vi "Get 7280 Formated Parameters.VI"(8 "error in (no error)":errorcluster, 10 "Initial String":string, 11 "VISA Resource Name":refnum<visa-resource-name>) -> (0 "error out":errorcluster, 1 "Sensitivity":dbl format="%.4e", 2 "Frequency":dbl format="%.2e", 3 "Parameters":string, 4 "Time Constant":dbl format="%.2e", 5 "Oscillator voltage":dbl format="%.2e", 6 "Data titles":string[](array[string])=["PE7280_Vx (V)", "PE7280_Vy (V)"], 7 "VISA Resource Name Out":refnum<visa-resource-name>)   [LabVIEW 2015]
uses:
  GPIB/VISA  Send Receive.vi
panel:
  out "Ref. phase":dbl format="%.2f"
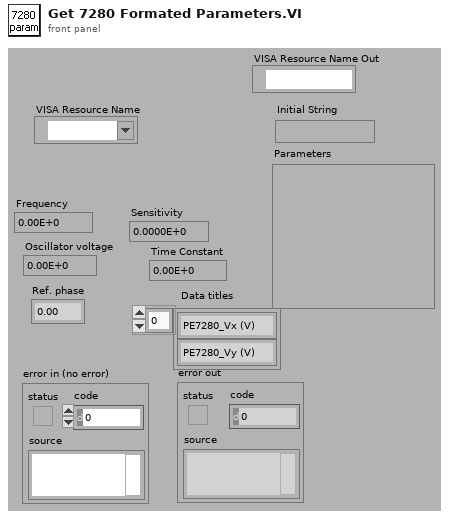
[diagram p1: front panel]
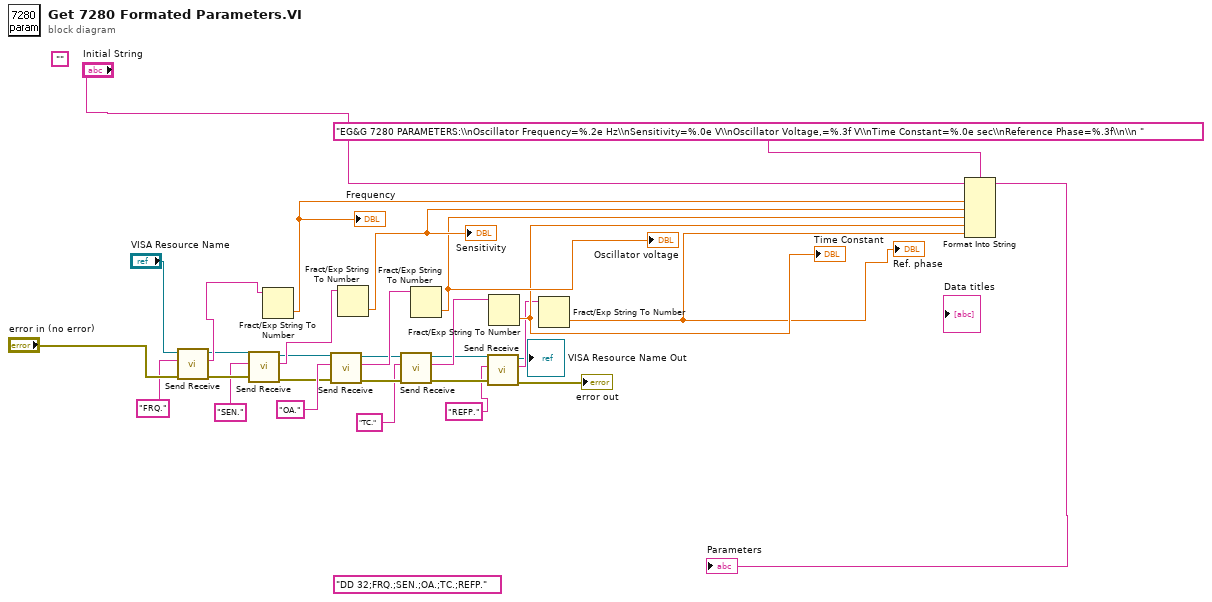
[diagram p0: block diagram]
diagram:
  (unwired) "DD 32;FRQ.;SEN.;OA.;TC.;REFP." ("data string")
  (unwired) ""
  n1 = call-poly "Send Receive.vi"("error in (no error)"="error in (no error)", "data string in"="FRQ." ("data string"), "VISA Resource Name"="VISA Resource Name") -> ("error out"=w19:errorcluster, "data string out"=w20:string, "VISA Resource Name Out"=w18:refnum<visa-resource-name>)  [unwired: 6 in]
  n2 = call-poly "Send Receive.vi"("error in (no error)"=w19, "data string in"="SEN." ("data string"), "VISA Resource Name"=w18) -> ("error out"=w14:errorcluster, "data string out"=w16:string, "VISA Resource Name Out"=w12:refnum<visa-resource-name>)  [unwired: 6 in]
  n3 = Fract/Exp String To Number(string=w20) -> (number=w26:dbl)  [unwired: 4 out]
  "Frequency" <- w26
  n4 = call-poly "Send Receive.vi"("error in (no error)"=w14, "data string in"="OA." ("data string"), "VISA Resource Name"=w12) -> ("error out"=w11:errorcluster, "data string out"=w13:string, "VISA Resource Name Out"=w10:refnum<visa-resource-name>)  [unwired: 6 in]
  n5 = Fract/Exp String To Number(string=w16) -> (number=w25:dbl)  [unwired: 4 out]
  "Sensitivity" <- w25
  n6 = call-poly "Send Receive.vi"("error in (no error)"=w11, "data string in"="TC." ("data string"), "VISA Resource Name"=w10) -> ("error out"=w7:errorcluster, "data string out"=w8:string, "VISA Resource Name Out"=w6:refnum<visa-resource-name>)  [unwired: 6 in]
  n7 = Fract/Exp String To Number(string=w13) -> (number=w24:dbl)  [unwired: 4 out]
  "Oscillator voltage" <- w24
  n8 = call-poly "Send Receive.vi"("error in (no error)"=w7, "data string in"="REFP." ("data string"), "VISA Resource Name"=w6) -> ("error out"=→"error out":errorcluster, "data string out"=w4:string, "VISA Resource Name Out"=→"VISA Resource Name Out":refnum<visa-resource-name>)  [unwired: 6 in]
  n9 = Fract/Exp String To Number(string=w8) -> (number=w23:dbl)  [unwired: 4 out]
  "Time Constant" <- w23
  n10 = Fract/Exp String To Number(string=w4) -> (number=w22:dbl)  [unwired: 4 out]
  "Ref. phase" <- w22
  n11 = Format Into String(format string="EG&G 7280 PARAMETERS:\\nOscillator Frequency=%.2e Hz\\nSensitivity=%.0e V\\nOscillator Voltage,=%.3f V\\nTime Constant=%.0e sec\\nReference Phase=%.3f\\n\\n ", initial string="Initial String", w26, w25, w24, w23, w22) -> (resulting string=→"Parameters":string)  [unwired: 1 in, 1 out]
